vi "RS_SMBV100A_CalculateLineScenario.vi"(8 "Start speed":dbl=10.0, 9 "acceleration":dbl, 10 "delta y":dbl=10.0, 11 "delta X":dbl=10.0) -> (2 "Finished Speed":dbl, 3 "Duration":dbl)   [LabVIEW 2018]
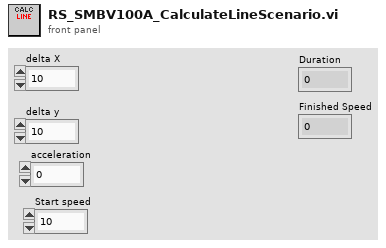
[diagram p1: front panel]
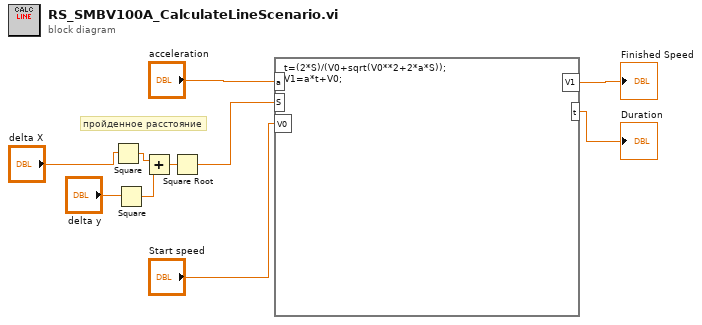
[diagram p0: block diagram]
diagram:
  # "пройденное расстояние"
  n1 = Square(x="delta X") -> (x^2=w9:dbl)
  n2 = Square(x="delta y") -> (x^2=w8:dbl)
  n3 = Add(x=w9, y=w8) -> (x+y=w10:dbl)
  n4 = Square Root(x=w10) -> (sqrt(x)=w3:dbl)
  n5 = formula code="t=(2*S)/(V0+sqrt(V0**2+2*a*S));\nV1=a*t+V0;"("a"="acceleration", "S"=w3, "V0"="Start speed") -> ("V1"=→"Finished Speed":dbl, "t"=→"Duration":dbl)
